vi "New Pod Coordinates.vi"(8 "Y translation":dbl=1.0 format="%#_13g", 9 "X translation":dbl=1.0 format="%#_13g", 11 "Radii (ft)":T2 {"Right Back Position" format="%.2f"; "Right Front Position" format="%.2f"; "Left Back Position" format="%.2f"; "Left Front Position" format="%.2f"}) -> (3 "output cluster":T1)   [LabVIEW 2020]
uses:
  Type Definitions/Data/Pod Positions.ctl
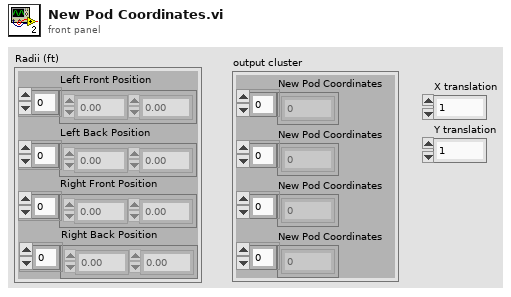
[diagram p1: front panel]
types:
  T1 = cluster{"New Pod Coordinates":dbl[], "New Pod Coordinates":dbl[], "New Pod Coordinates":dbl[], "New Pod Coordinates":dbl[]}
  T2 = typedef "Pod Positions.ctl" = cluster{"Left Front Position":dbl[], "Left Back Position":dbl[], "Right Front Position":dbl[], "Right Back Position":dbl[]}
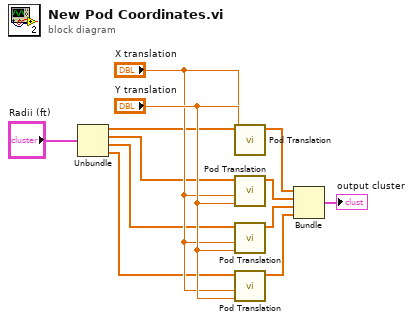
[diagram p0: block diagram]
diagram:
  n1 = Unbundle("Radii (ft)") -> ("Left Front Position"=w3:dbl[], "Left Back Position"=w4:dbl[], "Right Front Position"=w5:dbl[], "Right Back Position"=w6:dbl[])
  n2 = call "Pod Translation.vi"("Y translation"="Y translation", "X translation"="X translation", "Pod Coordinates"=w3) -> ("New Pod Coordinates"=w7:dbl[])  [unwired: 8 in]
  n3 = call "Pod Translation.vi"("Y translation"="Y translation", "X translation"="X translation", "Pod Coordinates"=w4) -> ("New Pod Coordinates"=w8:dbl[])  [unwired: 8 in]
  n4 = call "Pod Translation.vi"("Y translation"="Y translation", "X translation"="X translation", "Pod Coordinates"=w5) -> ("New Pod Coordinates"=w9:dbl[])  [unwired: 8 in]
  n5 = call "Pod Translation.vi"("Y translation"="Y translation", "X translation"="X translation", "Pod Coordinates"=w6) -> ("New Pod Coordinates"=w10:dbl[])  [unwired: 8 in]
  n6 = Bundle("New Pod Coordinates"=w7, "New Pod Coordinates"=w8, "New Pod Coordinates"=w9, "New Pod Coordinates"=w10) -> (→"output cluster":T1)  [unwired: 1 in]
